vi "Read Dark Color.vi"(8 "error in (no error)":errorcluster, 11 "BarCode in":refnum<class "BarCode.lvclass">) -> (0 "error out":errorcluster, 2 "Dark Color":u32(colorbox), 3 "BarCode out":refnum<class "BarCode.lvclass">)   [LabVIEW 2013, in "BarCodes.lvlib" / "BarCode.lvclass"]
doc: "Returns the dark color in the barcode. In typical barcodes, this is black"
uses:
  BarCode.lvclass
  BarCode.lvclass/BarCode.ctl
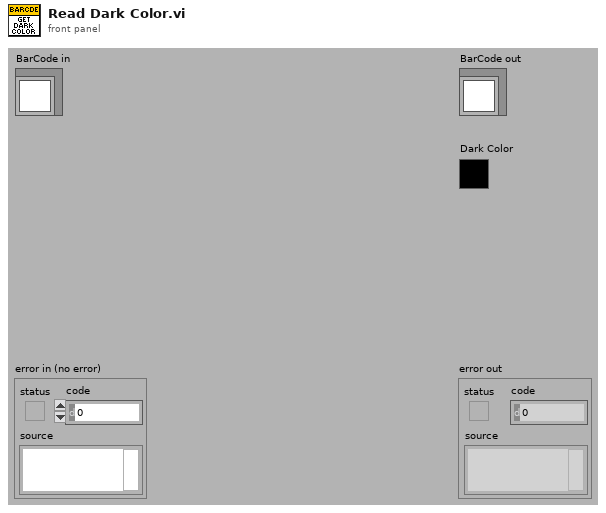
[diagram p1: front panel]
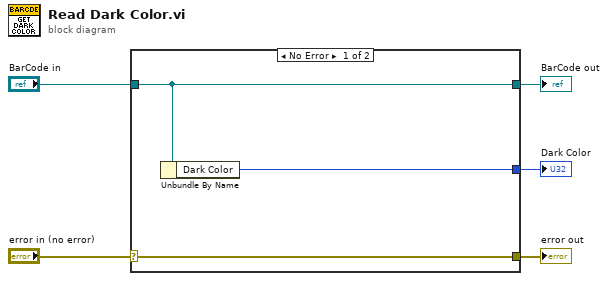
[diagram p0: block diagram]
diagram:
  n1 = case shown="No Error" "error in (no error)" {
    selector: "error in (no error)" -> [w8 w9]
    tunnel: [w8 w9] -> w4
    tunnel: [w7 w10] -> w2
    tunnel: "BarCode in" -> [w7 w10]
    tunnel: [w6 _] -> w1
    frame No Error {
      n2 = Unbundle By Name(w7) -> ("Dark Color"=w6:u32)
    }
    frame Error {
    }
  }
  "error out" <- w4
  "BarCode out" <- w2
  "Dark Color" <- w1
